vi "MergeFilesManual_Valise.vi"(4 "Error In":errorcluster, 7 "MergeFileConfINPUT":T1) -> (0 "sortie d'erreur":errorcluster)   [LabVIEW 2017]
uses:
  DefDeType/WhichPath.ctl
  DefDeType/MergeFileConfig.ctl
panel:
  out "MergeFileConfig":T1
  in  "Cancel":bool
  in  "OK Merge":bool
  out "AllWaveForms":waveform(dbl)[](graph)
  out "NortekWaveForms":waveform(dbl)[](graph)
  out "HexapodWaveForms":waveform(dbl)[](graph)
  out "QualisysWaveform":waveform(dbl)[](graph)
  out "ValiseWaveform":waveform(dbl)[](graph)
  out "Etat":string
  # "Merging files"
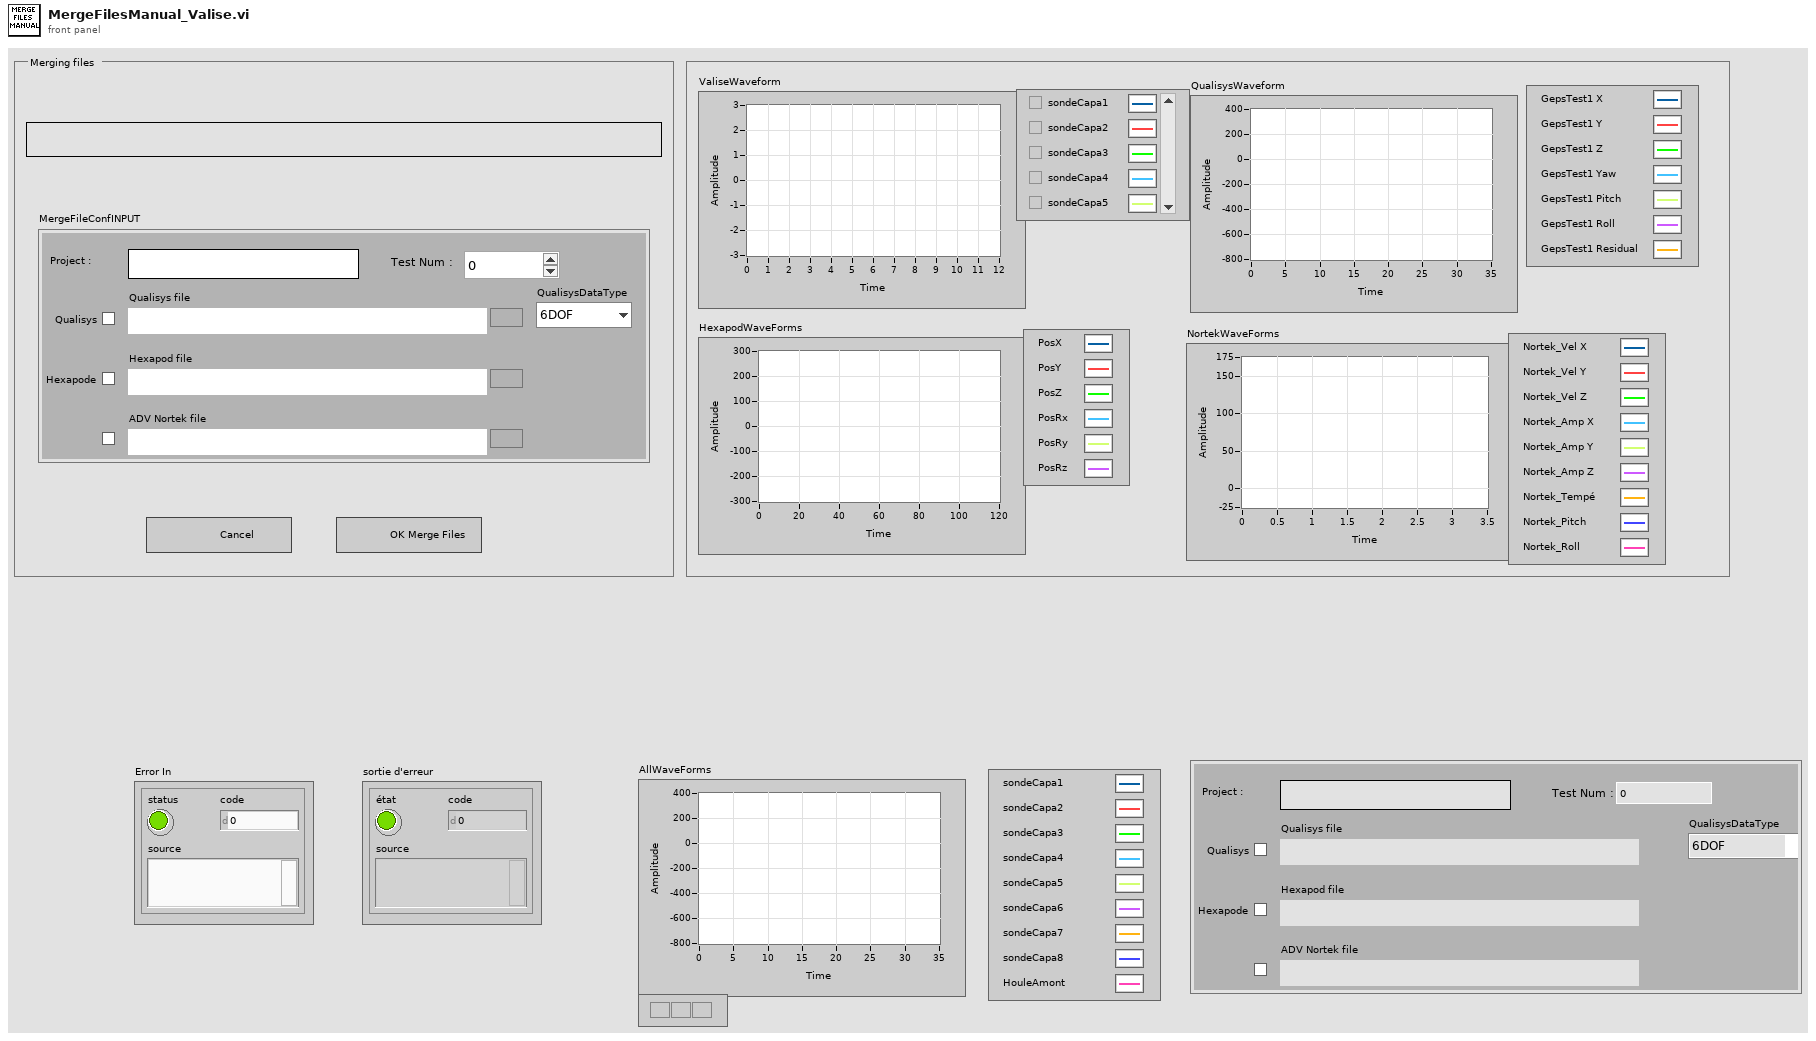
[diagram p1: front panel]
types:
  T1 = typedef "MergeFileConfig.ctl" = cluster{"Test Num : ":u32, "Project :":string, "Qualisys file":path, "Hexapod file":path, "ADV Nortek file":path, "QualisysDataType":enum16{"6DOF", "3DTracking", "6DOF + 3D"}, "Qualisys":bool, "Hexapode":bool, "ADV Nortek":bool}
  T2 = enum16{"open", "open or create", "create or replace", "create", "open (read-only)"}
  T3 = typedef "WhichPath.ctl" = enum16{"DossierProjet", "Config", "Meas", "MeasPCI", "MeasCRIO1", "MeasCRIO2", "MeasQualisys", "MeasHBM", "MeasTDMS", "Fig", "Res"}
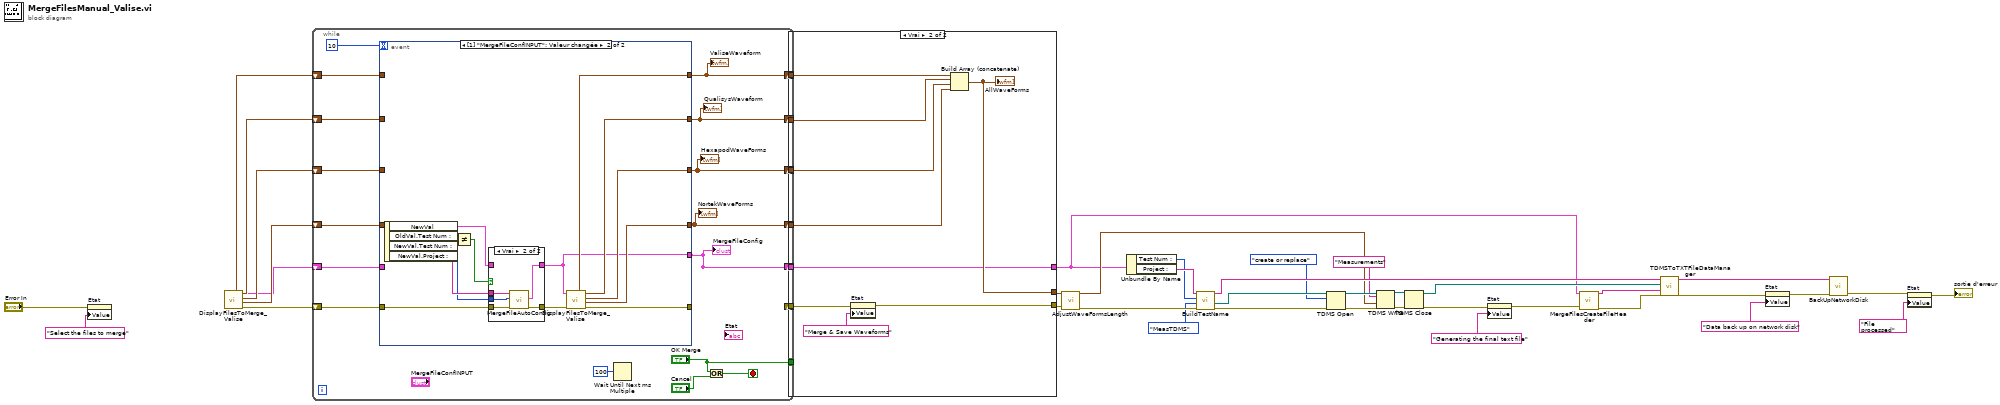
[diagram p0: block diagram]
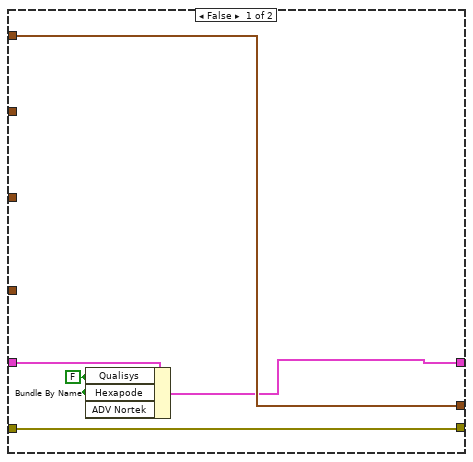
[diagram p2: hidden frame]
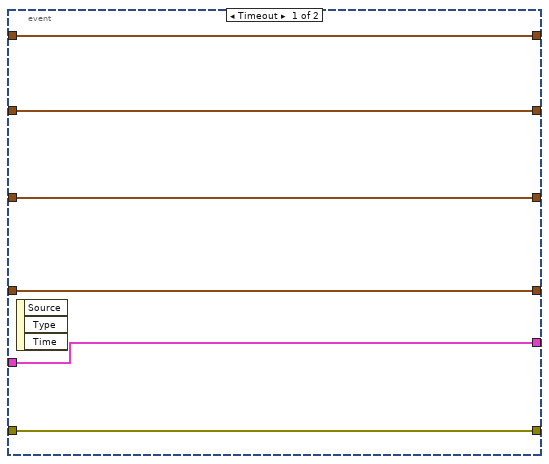
[diagram p3: hidden frame]
diagram:
  n1 = property on="Etat" class="Ch"(error in="Error In", "Value"="Select the files to merge" ("Etat")) -> (error out=w33:errorcluster)  [unwired: 1 in, 1 out]
  n2 = call "DisplayFilesToMerge_Valise.vi"() -> ("Error Out"=w41:errorcluster, "NortekWaveForms"=w36:waveform(dbl)[], "HexapodWaveForms"=w37:waveform(dbl)[], "QualisysWaveform"=w38:waveform(dbl)[], "ValiseWaveform"=w40:waveform(dbl)[], "Error In"=w39:errorcluster, "MergeFileConfigIN"=w2:T1)  [unwired: 3 in]
  n3 = while {
    shift-right: [w56] -> w43
    shift-left: w40 -> [w60]
    shift-right: [w55] -> w44
    shift-left: w38 -> [w59]
    shift-right: [w54] -> w45
    shift-left: w37 -> [w58]
    shift-right: [w53] -> w46
    shift-left: w36 -> [w57]
    shift-right: [w49] -> w42
    shift-left: w41 -> [w52]
    tunnel: ["OK Merge"] -> w5
    shift-right: [w48] -> w4
    shift-left: w2 -> [w50]
    stop <- w63 stop-if-true
    n4 = event shown="[1] \"MergeFileConfINPUT\": Valeur changée" {
      selector: _ -> [_ _]
      dyn-events: _ -> [_ _]
      timeout: 10 -> [_ _]
      tunnel: w60 -> [w70 _]
      tunnel: w59 -> [w69 _]
      tunnel: w58 -> [w68 _]
      tunnel: w57 -> [w67 _]
      tunnel: [w70 w82] -> w56
      tunnel: [w69 w81] -> w55
      tunnel: [w68 w80] -> w54
      tunnel: [w67 w79] -> w53
      tunnel: w52 -> [w66 w76]
      tunnel: [w66 w83] -> _
      tunnel: w50 -> [w65 _]
      tunnel: [w65 w71] -> w48
      event Timeout {
        n5 = event-data() -> ()  [unwired: 1 in, 3 out]
      }
      event Value Change {
        n6 = event-data() -> ("NewVal"=w72:T1, "OldVal.Test Num :"=w78:u32, "NewVal.Test Num :"=w73:u32, "NewVal.Project :"=w75:string)  [unwired: 1 in]
        n7 = Not Equal?(x=w78, y=w73) -> (x != y?=w74:bool)
        n8 = case shown="Vrai" w74 {
          tunnel: [w85 w89] -> w77
          tunnel: w76 -> [w85 w90]
          tunnel: w75 -> [_ w88]
          tunnel: w73 -> [_ w87]
          tunnel: w72 -> [w84 _]
          tunnel: [w84 w86] -> w71
          frame False {
          }
          frame True {
            n9 = call "MergeFileAutoConfig.vi"("error in (no error)"=w90, "test num"=w87, "ProjetIN"=w88) -> ("error out"=w89:errorcluster, "MergeFileConfigOUT"=w86:T1)  [unwired: 2 in, 1 out]
          }
        }
        n10 = call "DisplayFilesToMerge_Valise.vi"("Error In"=w77, "MergeFileConfigIN"=w71) -> ("Error Out"=w83:errorcluster, "NortekWaveForms"=w79:waveform(dbl)[], "HexapodWaveForms"=w80:waveform(dbl)[], "QualisysWaveform"=w81:waveform(dbl)[], "ValiseWaveform"=w82:waveform(dbl)[])  [unwired: 3 in]
      }
    }
    "ValiseWaveform" <- w56
    "QualisysWaveform" <- w55
    "HexapodWaveForms" <- w54
    "NortekWaveForms" <- w53
    "MergeFileConfig" <- w48
    n11 = Wait Until Next ms Multiple(millisecond multiple=u32 100) -> ()  [unwired: 1 out]
    n12 = Or(x="OK Merge", y="Cancel") -> (x .or. y?=w63:bool)
  }
  n13 = case shown="Vrai" w5 {
    tunnel: w46 -> [_ w104]
    tunnel: w45 -> [_ w103]
    tunnel: w44 -> [_ w102]
    tunnel: w43 -> [w94 w101]
    tunnel: w42 -> [w95 w100]
    tunnel: [w94 w99] -> w15
    tunnel: [w95 w97] -> w13
    tunnel: w4 -> [w93 w96]
    tunnel: [w91 w96] -> w3
    frame False {
      w92 = FALSE ("Qualisys")
      n14 = Bundle By Name(cluster=w93, "Qualisys"=w92, "Hexapode"=w92, "ADV Nortek"=w92) -> (w91:T1)
    }
    frame True {
      n15 = property on="Etat" class="Ch"(error in=w100, "Value"="Merge & Save Waveforms" ("Etat")) -> (error out=w97:errorcluster)  [unwired: 1 in, 1 out]
      n16 = Build Array (concatenate)(w101, w102, w103, w104) -> (w99:waveform(dbl)[])
      "AllWaveForms" <- w99
    }
  }
  n17 = call "AdjustWaveFormsLength.vi"("error in (no error)"=w13, "AllWaveFormsIN"=w15) -> ("error out"=w25:errorcluster, "AllWaveFormsOUT"=w11:waveform(dbl)[])  [unwired: 4 in]
  n18 = Unbundle By Name(w3) -> ("Test Num :"=w9:u32, "Project :"=w10:string)
  n19 = call "BuildTestName.vi"("entrée d'erreur"=w25, "WhichPath?"=WhichPath."MeasTDMS", "NextTestNum"=w9, "NomProjet"=w10) -> ("sortie d'erreur"=w22:errorcluster, "cheminProchainFichier"=w19:path, "NomProjetOut"=w24:string)  [unwired: 1 in, 1 out]
  n20 = TDMS Open(8:w22, 10:T2."create or replace" ("operation (0:open)"), 11:w19) -> (0:w21:errorcluster, 3:w17:refnum<k34>)  [unwired: 4 in]
  n21 = TDMS Write(0:w17, 5:"Measurements" ("group name in (Untitled)"), 9:w11, 11:w21) -> (4:w16:refnum<k34>, 15:w20:errorcluster)  [unwired: 2 in, 2 out]
  n22 = TDMS Close(8:w20, 11:w16) -> (0:w14:errorcluster, 3:w12:path)
  n23 = property on="Etat" class="Ch"(error in=w14, "Value"="Generating the final text file" ("Etat")) -> (error out=w8:errorcluster)  [unwired: 1 in, 1 out]
  n24 = call "MergeFilesCreateFileHeader.vi"("Error In"=w8, "MergeFileConfig"=w3) -> ("Error Out"=w7:errorcluster, "TextFileHeader"=w6:string)  [unwired: 4 in]
  n25 = call "TDMSToTXTFileDataManager.vi"("entrée d'erreur"=w7, "Info(analog acq,wave,Quali,hexap...)"=w6, "FichierTDMSOrigine"=w12, "NomProj"=w24) -> ("sortie d'erreur"=w29:errorcluster, "NomProjOUT"=w28:string)  [unwired: 1 in, 1 out]
  n26 = property on="Etat" class="Ch"(error in=w29, "Value"="Data back up on network disk" ("Etat")) -> (error out=w30:errorcluster)  [unwired: 1 in, 1 out]
  n27 = call "BackUpNetworkDisk.vi"("Entrée d'erreur"=w30, "NomProjet"=w28) -> ("error out"=w27:errorcluster)  [unwired: 2 in, 1 out]
  n28 = property on="Etat" class="Ch"(error in=w27, "Value"="File processed" ("Etat")) -> (error out=→"sortie d'erreur":errorcluster)  [unwired: 1 in, 1 out]
